vi "Log Framework Event.vi"(7 "Event Level (Debug)":T1, 8 "error in (no error)":errorcluster, 9 "Data To Log":string, 10 "Caller Info (\"\")":string, 11 "Topic In":refnum<class "Topic.lvclass">) -> (0 "error out":errorcluster)   [LabVIEW 2017, in "Mediator.lvlib" / "Topic.lvclass"]
uses:
  Topic.lvclass
  gpm_packages/@cs/event-logger/Source/Composed Log/Types/Log Level.ctl
  Topic.lvclass/Topic.ctl
  gpm_packages/@cs/event-logger/Source/Composed Log/LoggerReference/LoggerReference.lvclass/LoggerReference.ctl
  gpm_packages/@cs/event-logger/Source/Composed Log/LoggerReference/Log.vi
  gpm_packages/@cs/event-logger/Source/Composed Log/LoggerReference/Get Valid Event Time.vi
  gpm_packages/@cs/event-logger/Source/Composed Log/LoggerReference/Remove Stale Logs.vi
  gpm_packages/@cs/event-logger/Source/Composed Log/LoggerReference/LoggerReference.lvclass
  gpm_packages/@cs/event-logger/Source/Composed Log/Composed Log.lvlib
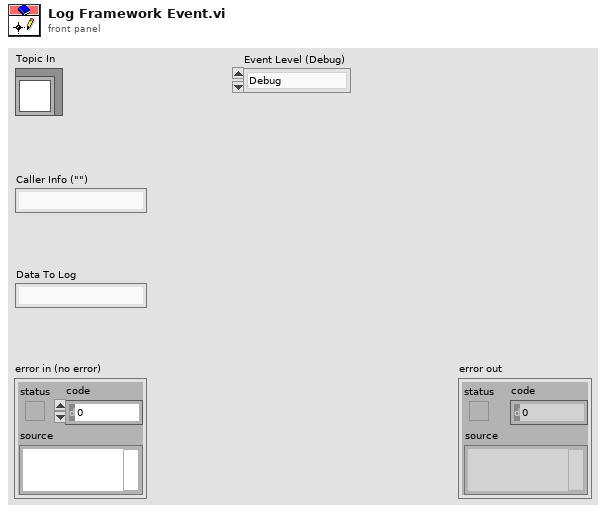
[diagram p1: front panel]
types:
  T1 = typedef "Composed Log.lvlib/Log Level.ctl" = enum16{"Debug", "Info", "Warning", "Error", "Critical"}
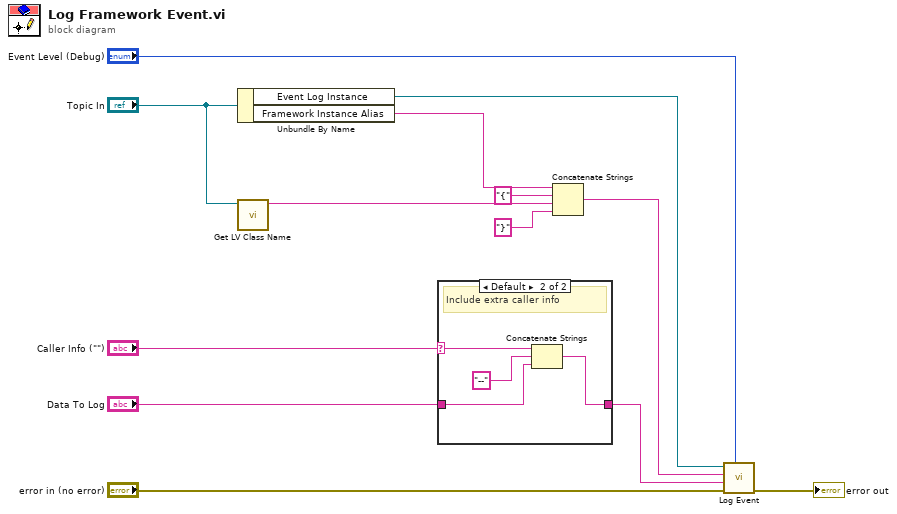
[diagram p0: block diagram]
diagram:
  n1 = Unbundle By Name("Topic In") -> ("Event Log Instance"=w11:refnum<class "LoggerReference.lvclass">, "Framework Instance Alias"=w9:string)
  n2 = call <vilib>:"Get LV Class Name.vi"("object"="Topic In") -> ("class name"=w6:string)  [unwired: 9 in, 1 out]
  n3 = case shown="Default" "Caller Info (\"\")" {
    selector: "Caller Info (\"\")" -> [_ w18]
    tunnel: "Data To Log" -> [w14 w15]
    tunnel: [w14 w16] -> w1
    frame "" {
      # "No additional info"
    }
    frame Default {
      # "Include extra caller info"
      n4 = Concatenate Strings(w18, "--" ("string"), w15) -> (w16:string)
    }
  }
  n5 = Concatenate Strings(w9, "{" ("string"), w6, "}" ("string")) -> (w8:string)
  n6 = call "Log Event.vi"("Event Level"="Event Level (Debug)", "error in (no error)"="error in (no error)", "Data To Log"=w1, "SourceID"=w8, "Log Instance"=w11) -> ("error out"=→"error out":errorcluster)  [unwired: 5 in, 1 out]
